vi "FT_Search All (ver 2).vi"(8 "error in (no error)":errorcluster, 11 "CTA Test#":string="CTA013A") -> (0 "error Out":errorcluster, 2 "All FT":T1(array[cluster]), 3 "Select Ft":T2)   [LabVIEW 2009]
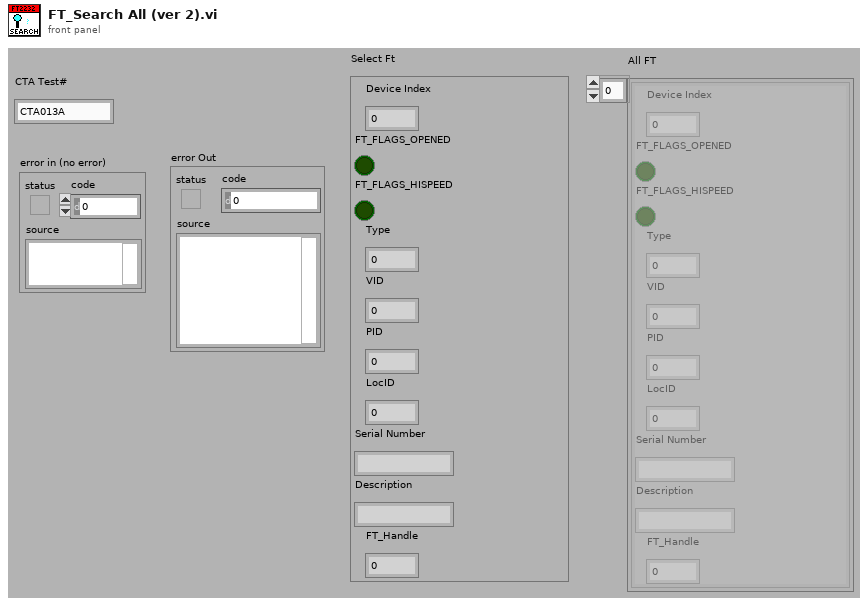
[diagram p1: front panel]
types:
  T1 = cluster{"Device Index":u32, "FT_FLAGS_OPENED":bool, "FT_FLAGS_HISPEED":bool, "Type":u32, "VID":u32, "PID":u32, "LocID":i32, "Serial Number":string, "Description":string, "FT_Handle":u32}[]
  T2 = cluster{"Device Index":u32, "FT_FLAGS_OPENED":bool, "FT_FLAGS_HISPEED":bool, "Type":u32, "VID":u32, "PID":u32, "LocID":i32, "Serial Number":string, "Description":string, "FT_Handle":u32}
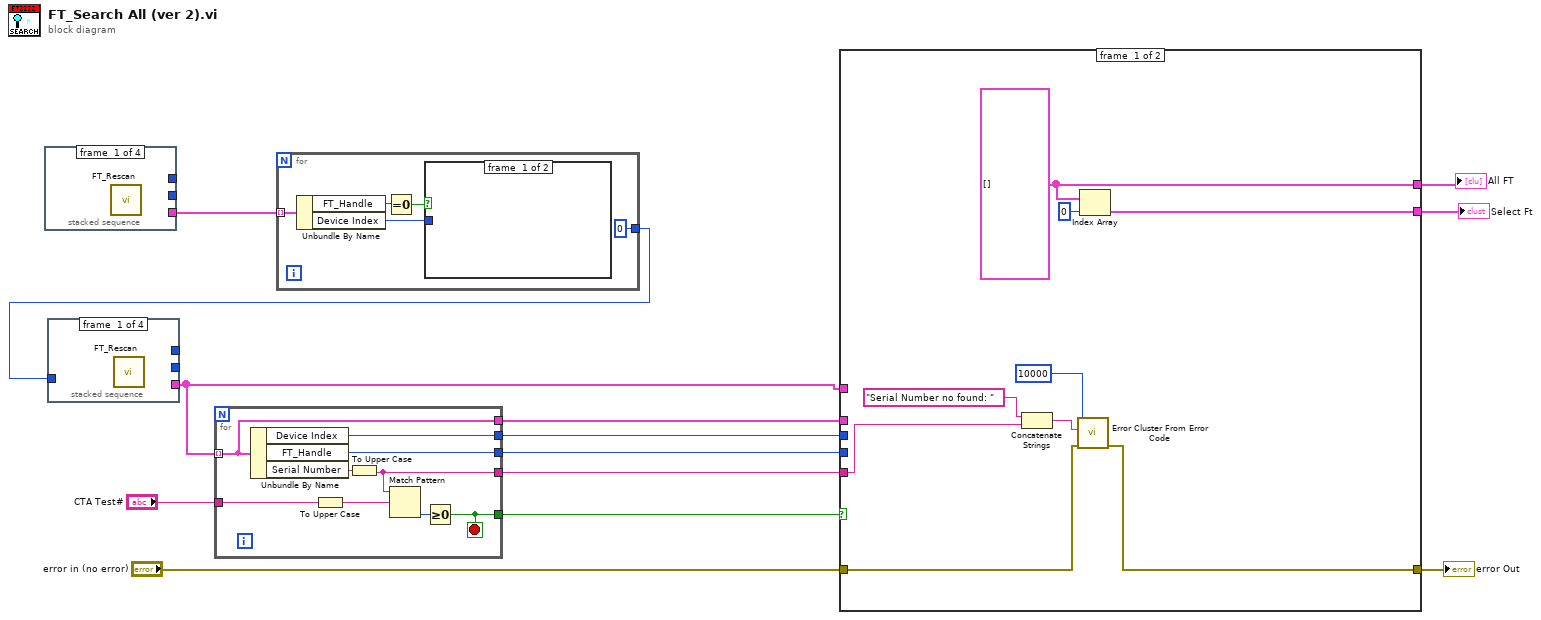
[diagram p0: block diagram]
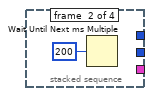
[diagram p2: hidden frame]
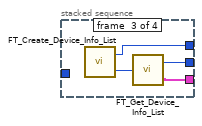
[diagram p3: hidden frame]
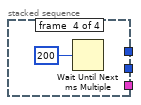
[diagram p4: hidden frame]
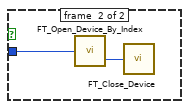
[diagram p5: hidden frame]
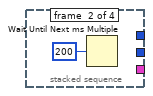
[diagram p6: hidden frame]
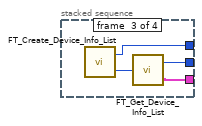
[diagram p7: hidden frame]
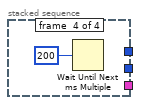
[diagram p8: hidden frame]
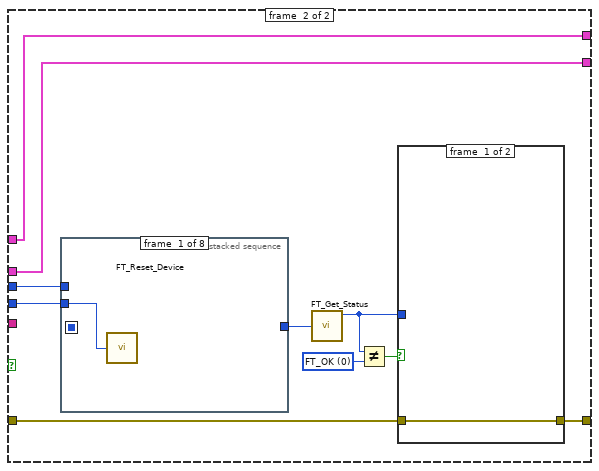
[diagram p9: hidden frame]
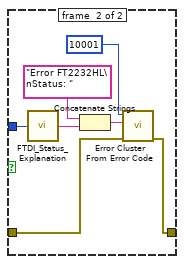
[diagram p10: hidden frame]
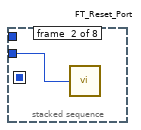
[diagram p11: hidden frame]
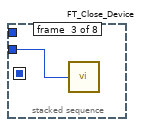
[diagram p12: hidden frame]
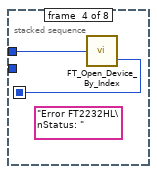
[diagram p13: hidden frame]
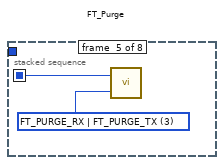
[diagram p14: hidden frame]
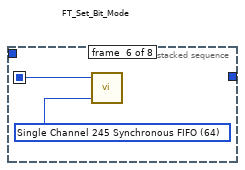
[diagram p15: hidden frame]
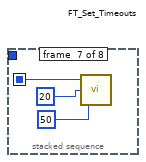
[diagram p16: hidden frame]
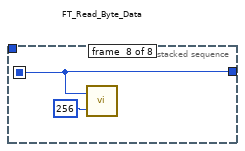
[diagram p17: hidden frame]
diagram:
  n1 = stacked-sequence {
    tunnel: [_ _ w17 _] -> w3
    tunnel: [_ _ w16 _] -> _
    tunnel: [_ _ w15 _] -> _
    frame #0 {
      n2 = call "FT_Rescan.vi"() -> ()  [unwired: 1 in, 1 out]
    }
    frame #1 {
      n3 = Wait Until Next ms Multiple(millisecond multiple=u32 200) -> ()  [unwired: 1 out]
    }
    frame #2 {
      n4 = call "FT_Create_Device_Info_List.vi"() -> ("Number of Devices"=w18:u32, "FT_Status"=w16:u32)
      n5 = call "FT_Get_Device_Info_List.vi"("Number Of Devices"=w18) -> ("FT_Status"=w15:u32, "Device Info List"=w17:T1)
    }
    frame #3 {
      n6 = Wait Until Next ms Multiple(millisecond multiple=u32 200) -> ()  [unwired: 1 out]
    }
  }
  n7 = for {
    tunnel: w3 -> [w24] mode=indexing
    tunnel: [u32 0 ("FT_Status")] -> w2
    n8 = Unbundle By Name(w24) -> ("FT_Handle"=w23:u32, "Device Index"=w22:u32)
    n9 = Equal To 0?(x=w23) -> (x = 0?=w21:bool)
    n10 = case shown="True" w21 {
      tunnel: w22 -> [_ w26]
      frame #0 {
      }
      frame #1 {
        n11 = call "FT_Open_Device_By_Index.vi"("Device Index"=w26) -> ("Handle"=w25:u32)  [unwired: 1 out]
        n12 = call "FT_Close_Device.vi"("Handle"=w25) -> ()  [unwired: 1 out]
      }
    }
  }
  n13 = stacked-sequence {
    tunnel: [_ _ w30 _] -> w1
    tunnel: [_ _ w29 _] -> _
    tunnel: [_ _ w28 _] -> _
    tunnel: w2 -> [_ _ _ _]
    frame #0 {
      n14 = call "FT_Rescan.vi"() -> ()  [unwired: 1 in, 1 out]
    }
    frame #1 {
      n15 = Wait Until Next ms Multiple(millisecond multiple=u32 200) -> ()  [unwired: 1 out]
    }
    frame #2 {
      n16 = call "FT_Create_Device_Info_List.vi"() -> ("Number of Devices"=w31:u32, "FT_Status"=w29:u32)
      n17 = call "FT_Get_Device_Info_List.vi"("Number Of Devices"=w31) -> ("FT_Status"=w28:u32, "Device Info List"=w30:T1)
    }
    frame #3 {
      n18 = Wait Until Next ms Multiple(millisecond multiple=u32 200) -> ()  [unwired: 1 out]
    }
  }
  n19 = for {
    tunnel: w1 -> [w34] mode=indexing
    tunnel: "CTA Test#" -> [w39]
    tunnel: [w37] -> w4
    tunnel: [w36] -> w12
    tunnel: [w35] -> w11
    tunnel: [w34] -> w7
    tunnel: [w33] -> w5
    stop <- w37 stop-if-true
    n20 = Unbundle By Name(w34) -> ("Device Index"=w36:u32, "FT_Handle"=w35:u32, "Serial Number"=w40:string)
    n21 = To Upper Case(1:w39) -> (0:w38:string)
    n22 = To Upper Case(1:w40) -> (0:w33:string)
    n23 = Match Pattern(string=w33, regular expression=w38) -> (offset past match=w41:i32)  [unwired: 4 out]
    n24 = Greater Or Equal To 0?(x=w41) -> (x >= 0?=w37:bool)
  }
  n25 = case shown="True" w4 {
    tunnel: w1 -> [_ w58]
    tunnel: w12 -> [_ w60]
    tunnel: w11 -> [_ w59]
    tunnel: "error in (no error)" -> [w48 w52]
    tunnel: [w47 w51] -> w9
    tunnel: [w44 w57] -> w6
    tunnel: [w45 w58] -> w8
    tunnel: w7 -> [_ w57]
    tunnel: w5 -> [w43 _]
    frame #0 {
      w45 = T1 [] ("All FT")
      n26 = Concatenate Strings("Serial Number no found: ", w43) -> (w49:string)
      n27 = call <vilib>:"Error Cluster From Error Code.vi"("error in (no error)"=w48, "error message (\"\")"=w49, "error code (0)"=10000 ("error code (no error:0)")) -> ("error out"=w47:errorcluster)  [unwired: 1 in, 5 out]
      n28 = Index Array(array=w45, index=0) -> (element=w44:T2)
    }
    frame #1 {
      w55 = u32 0 items=["FT_OK", "FT_INVALID_HANDLE", "FT_DEVICE_NOT_FOUND", "FT_DEVICE_NOT_OPENED", "FT_IO_ERROR", "FT_INSUFFICIENT_RESOURCES", "FT_INVALID_PARAMETER", "FT_INVALID_BAUD_RATE", "FT_DEVICE_NOT_OPENED_FOR_ERASE", "FT_DEVICE_NOT_OPENED_FOR_WRITE", "FT_FAILED_TO_WRITE_DEVICE", "FT_EEPROM_READ_FAILED", "FT_EEPROM_WRITE_FAILED", "FT_EEPROM_ERASE_FAILED", "FT_EEPROM_NOT_PRESENT", "FT_EEPROM_NOT_PROGRAMMED", "FT_INVALID_ARGS", "FT_NOT_SUPPORTED", "FT_OTHER_ERROR"] ("FT_Status")
      n29 = stacked-sequence {
        seq-local: [_ _ _ w72 _ _ _ _] -> [_ _ _ _ w74 w76 w78 w81]
        tunnel: w59 -> [w69 w70 w71 _ _ _ _ _]
        tunnel: w60 -> [_ _ _ w73 _ _ _ _]
        tunnel: [_ _ _ _ _ _ _ w81] -> w56
        frame #0 {
          n30 = call "FT_Reset_Device.vi"("Handle"=w69) -> ()  [unwired: 1 out]
        }
        frame #1 {
          n31 = call "FT_Reset_Port.vi"("Handle"=w70) -> ()  [unwired: 1 out]
        }
        frame #2 {
          n32 = call "FT_Close_Device.vi"("Handle"=w71) -> ()  [unwired: 1 out]
        }
        frame #3 {
          (unwired) "Error FT2232HL\nStatus: "
          n33 = call "FT_Open_Device_By_Index.vi"("Device Index"=w73) -> ("Handle"=w72:u32)  [unwired: 1 out]
        }
        frame #4 {
          w75 = u32 3 items=["FT_PURGE_RX"=1, "FT_PURGE_TX"=2, "FT_PURGE_RX | FT_PURGE_TX"=3] ("Purge Flags")
          n34 = call "FT_Purge.vi"("Purge Flags"=w75, "Handle"=w74) -> ()  [unwired: 1 out]
        }
        frame #5 {
          w77 = u8 64 items=["Reset Bit Mode"=0, "Asynchronous Bit Bang"=1, "MPSSE"=2, "Synchronous Bit Bang"=4, "MCU Host Bus Emulation"=8, "Fast Opto-Isolated Serial"=16, "CBUS Bit Bang"=32, "Single Channel 245 Synchronous FIFO"=64] ("Bit Mode")
          n35 = call "FT_Set_Bit_Mode.vi"("Bit Mode"=w77, "Handle"=w76) -> ()  [unwired: 1 in, 1 out]
        }
        frame #6 {
          n36 = call "FT_Set_Timeouts.vi"("Write Timeout"=u32 50, "Read Timeout"=u32 20, "Handle"=w78) -> ()  [unwired: 1 out]
        }
        frame #7 {
          n37 = call "FT_Read_Byte_Data.vi"("Handle"=w81, "Bytes To Read"=u32 256) -> ()  [unwired: 3 out]
        }
      }
      n38 = call "FT_Get_Status.vi"("Handle"=w56) -> ("FT_Status"=w53:u32)  [unwired: 3 out]
      n39 = Not Equal?(x=w53, y=w55) -> (x != y?=w54:bool)
      n40 = case shown="False" w54 {
        tunnel: w53 -> [_ w68]
        tunnel: w52 -> [w61 w65]
        tunnel: [w61 w64] -> w51
        frame #0 {
        }
        frame #1 {
          n41 = call "FTDI_Status_Explanation.vi"("FT_Status"=w68) -> ("Status String"=w67:string)
          n42 = Concatenate Strings("Error FT2232HL\nStatus: ", w67) -> (w62:string)
          n43 = call <vilib>:"Error Cluster From Error Code.vi"("error in (no error)"=w65, "error message (\"\")"=w62, "error code (0)"=10001 ("error code (no error:0)")) -> ("error out"=w64:errorcluster)  [unwired: 1 in, 5 out]
        }
      }
    }
  }
  "Select Ft" <- w6
  "error Out" <- w9
  "All FT" <- w8
